vi "Spaltenindex finden.vi"(10 "Tabelle":string[][](array[string]), 11 "Regulärer Ausdruck":string) -> (2 "Tab Zeile":i32, 3 "Tab Spalte":i32)   [LabVIEW 2015, in "Sprachverwaltung.lvlib"]
uses:
  Sprachverwaltung.lvlib
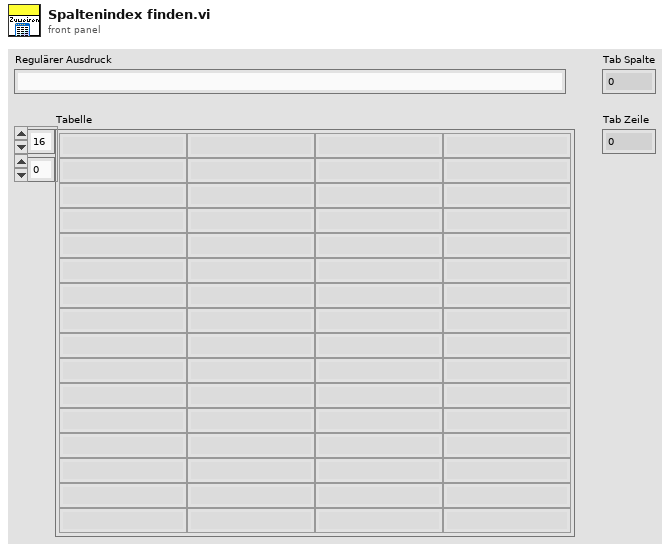
[diagram p1: front panel]
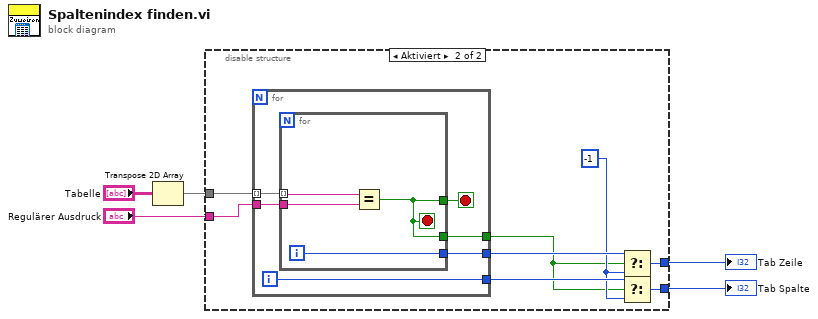
[diagram p0: block diagram]
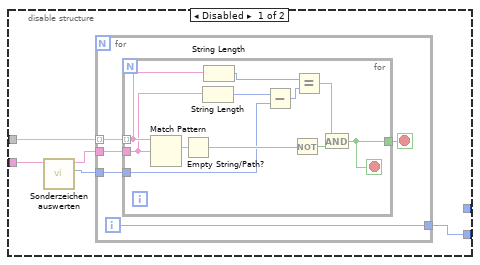
[diagram p2: hidden frame]
diagram:
  n1 = Transpose 2D Array(2D array="Tabelle") -> (transposed array=w3:string[][])
  n2 = disable-structure shown="Aktiviert" {
    disable-tunnel: [w9 w28] -> w4
    disable-tunnel: w3 -> [w8 w33]
    disable-tunnel: "Regulärer Ausdruck" -> [w7 w34]
    disable-tunnel: [_ w29] -> w1
    frame Disabled {
      n3 = call "Sonderzeichen auswerten.vi"("String"=w7) -> ("Anzahl"=w6:i32, "Suchstring"=w10:string)  [unwired: 9 in]
      n4 = for {
        tunnel: w10 -> [w15]
        tunnel: w8 -> [w14] mode=indexing
        tunnel: [w12] -> w9
        tunnel: w6 -> [w11]
        i -> [w12]
        stop <- w13 stop-if-true
        n5 = for {
          tunnel: w15 -> [w23]
          tunnel: w14 -> [w24] mode=indexing
          tunnel: [w18] -> w13
          tunnel: w11 -> [w16]
          stop <- w18 stop-if-true
          n6 = Match Pattern(string=w24, regular expression=w23) -> (match substring=w26:string)  [unwired: 1 in, 3 out]
          n7 = Empty String/Path?(string/path=w26) -> (empty?=w25:bool)
          n8 = String Length(string=w23) -> (length=w21:i32)
          n9 = String Length(string=w24) -> (length=w22:i32)
          n10 = Subtract(x=w21, y=w16) -> (x-y=w17:i32)
          n11 = Not(x=w25) -> (.not. x?=w20:bool)
          n12 = Equal?(x=w22, y=w17) -> (x = y?=w19:bool)
          n13 = And(x=w19, y=w20) -> (x .and. y?=w18:bool)
        }
      }
    }
    frame Enabled {
      w30 = -1 ("t")
      n14 = for {
        tunnel: w34 -> [w40]
        tunnel: w33 -> [w39] mode=indexing
        tunnel: [w37] -> w31
        tunnel: [w36] -> w32
        tunnel: [w35] -> w27
        i -> [w37]
        stop <- w38 stop-if-true
        n15 = for {
          tunnel: w40 -> [w43]
          tunnel: w39 -> [w44] mode=indexing
          tunnel: [w41] -> w38
          tunnel: [w42] -> w36
          tunnel: [w41] -> w35
          i -> [w42]
          stop <- w41 stop-if-true
          n16 = Equal?(x=w44, y=w43) -> (x = y?=w41:bool)
        }
      }
      n17 = Select(t=w32, s=w27, f=w30) -> (s? t:f=w29:i32)
      n18 = Select(t=w31, s=w27, f=w30) -> (s? t:f=w28:i32)
    }
  }
  "Tab Spalte" <- w4
  "Tab Zeile" <- w1
